vi "Parse Modbus Data.vi"(10 "Start Index":i32, 11 "Register Data":u16[](array[numeric])) -> (3 "Result":dbl)   [LabVIEW 2021]
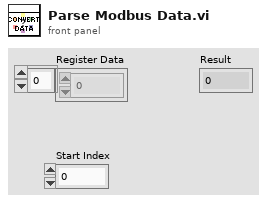
[diagram p1: front panel]
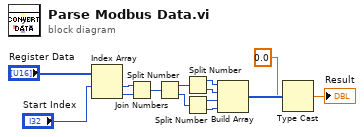
[diagram p0: block diagram]
diagram:
  n1 = Index Array(array="Register Data", index #1="Start Index") -> (element #1=w12:u16, element #2=w11:u16)  [unwired: 1 in]
  n2 = Join Numbers(hi=w12, lo=w11) -> ((hi.lo)=w10:u32)
  n3 = Split Number(x=w10) -> (hi(x)=w2:u16, lo(x)=w1:u16)
  n4 = Split Number(x=w2) -> (hi(x)=w9:u8, lo(x)=w8:u8)
  n5 = Split Number(x=w1) -> (hi(x)=w7:u8, lo(x)=w6:u8)
  n6 = Build Array(w9, w8, w7, w6) -> (w5:u8[])
  n7 = Type Cast(type=sgl 0.0 ("number"), x=w5) -> (*(type *) &x=→"Result":sgl)
